vi "axex_cell_xy_to_name.vi"(0 "cell xy in":T1, 1 "xy indexing from 1 (False)":bool) -> (2 "cell xy out":T1, 3 "cell name":string, 4 "column":i32, 5 "row":i32)   [LabVIEW 2020, in "AX Excel.lvlib"]
doc: "Call this to convert [x,y] cell coordinates to cell name (A1, BV5, ...) or to convert cell name to coordinates. \nIf input cell name is specified, the name will be converted to [x,y] coordinates.\nIf input cell name is empty, the coordinates will be converted to the cell name.\n\nOptionally you can select [x,y] indexing from 1 instead of 0."
uses:
  AX Excel.lvlib
  axex_cell_xy.ctl
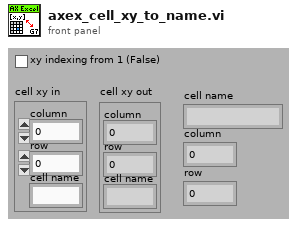
[diagram p1: front panel]
types:
  T1 = typedef "AX Excel.lvlib/axex_cell_xy.ctl" = cluster{"column":i32, "row":i32, "cell name":string}
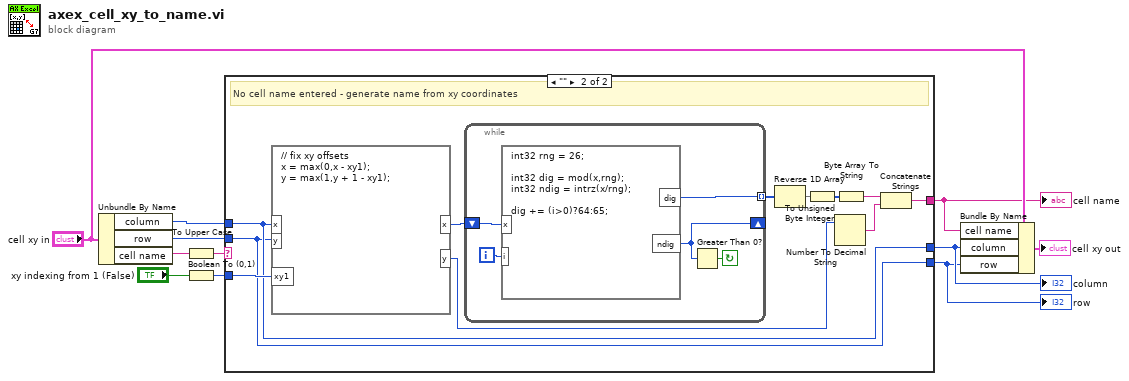
[diagram p0: block diagram]
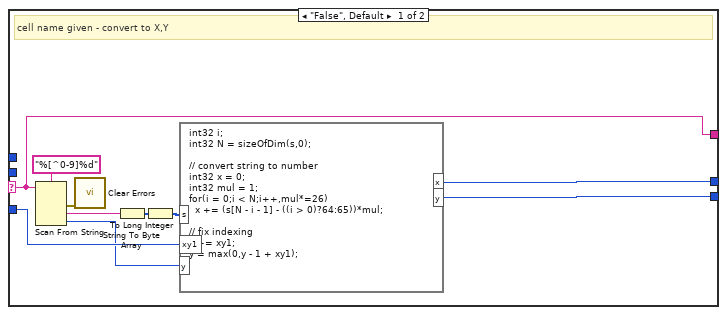
[diagram p2: hidden frame]
diagram:
  n1 = Unbundle By Name("cell xy in") -> ("column"=w9:i32, "row"=w10:i32, "cell name"=w11:string)
  n2 = To Upper Case(1:w11) -> (0:w7:string)
  n3 = Boolean To (0,1)(Boolean="xy indexing from 1 (False)") -> (0, 1=w6:i16)
  n4 = case shown="\"\"" w7 {
    selector: w7 -> [w14 _]
    tunnel: w10 -> [_ w22]
    tunnel: w9 -> [_ w23]
    tunnel: w6 -> [w17 w24]
    tunnel: [w14 w25] -> w3
    tunnel: [w13 w23] -> w4
    tunnel: [w12 w22] -> w1
    frame "False", Default {
      # "cell name given - convert to X,Y"
      n5 = Scan From String(format string="%[^0-9]%d", input string=w14) -> (error out=w15:errorcluster, output 1=w20:string, output 2=w16:i32)  [unwired: 4 in, 2 out]
      n6 = call <vilib>:"Clear Errors.vi"("error in (no error)"=w15) -> ()  [unwired: 5 in, 2 out]
      n7 = String To Byte Array(string=w20) -> (unsigned byte array=w19:u8[])
      n8 = To Long Integer(number=w19) -> (32bit integer=w18:i32[])
      n9 = formula code="int32 i;\nint32 N = sizeOfDim(s,0);\n\n// convert string to number\nint32 x = 0;\nint32 mul = 1;\nfor(i = 0;i < N;i++,mul*=26)\n  x += (s[N - i - 1] - ((i > 0)?64:65))*mul;\n\n// fix indexing\nx += xy1;\ny = max(0,y - 1 + xy1);"("s"=w18, "xy1"=w17, "y"=w16) -> ("x"=w13:i32, "y"=w12:i32)
    }
    frame "" {
      # "No cell name entered - generate name from xy coordinates"
      n10 = formula code="// fix xy offsets\nx = max(0,x - xy1);\ny = max(1,y + 1 - xy1);"("y"=w22, "x"=w23, "xy1"=w24) -> ("x"=w32:i32, "y"=w28:i32)
      n11 = while {
        shift-right: [w35] -> _
        shift-left: w32 -> [w37]
        tunnel: [w34] -> w30 mode=indexing
        i -> [w33]
        stop <- w36 continue-if-true
        n12 = formula code="int32 rng = 26;\n\nint32 dig = mod(x,rng);\nint32 ndig = intrz(x/rng);\n\ndig += (i>0)?64:65;"("x"=w37, "i"=w33) -> ("dig"=w34:i32, "ndig"=w35:i32)
        n13 = Greater Than 0?(x=w35) -> (x > 0?=w36:bool)
      }
      n14 = Reverse 1D Array(array=w30) -> (reversed array=w29:i32[])
      n15 = To Unsigned Byte Integer(number=w29) -> (unsigned 8bit integer=w31:u8[])
      n16 = Number To Decimal String(number=w28) -> (decimal integer string=w26:string)  [unwired: 1 in]
      n17 = Byte Array To String(unsigned byte array=w31) -> (string=w27:string)
      n18 = Concatenate Strings(w27, w26) -> (w25:string)
    }
  }
  "cell name" <- w3
  "column" <- w4
  "row" <- w1
  n19 = Bundle By Name(cluster="cell xy in", "cell name"=w3, "column"=w4, "row"=w1) -> (→"cell xy out":T1)
